vi "Desktop Main.vi"() -> ()   [LabVIEW 2017]
doc: "Demonstrates how to read the button value of the myRIO from the Shared Variable node."
panel:
  out "Boolean 2":bool
  out "error out":errorcluster
  in  "Stop":bool
  # "Overview: Demonstrates how to read the button value of the myRIO from the Shared Variable node.\nInstructions:\n1. Ensure RT Main.vi is already running.\n2. Run this VI. \n3. Press the user button on the myRIO device as many times as you want and observe the value changes of the Button indicator on this VI.\n4. Click Stop to stop this VI."
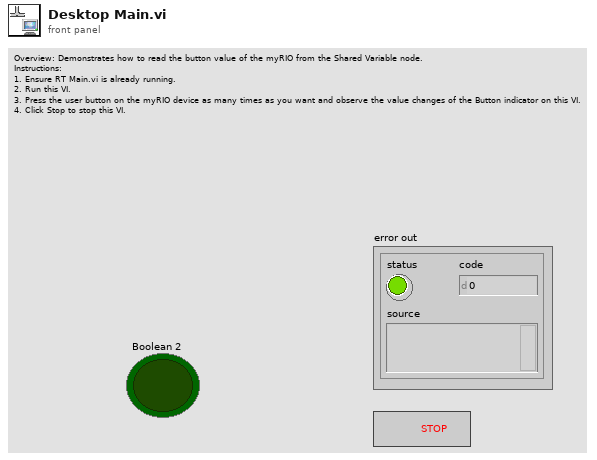
[diagram p1: front panel]
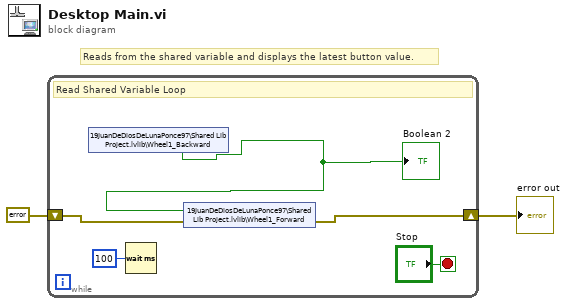
[diagram p0: block diagram]
diagram:
  # "Reads from the shared variable and displays the latest button value."
  n1 = while {
    shift-right: [w4] -> w1
    shift-left: errorcluster {"status"=FALSE, "code"=0, "source"=""} ("error in (no error)") -> [w5]
    stop <- "Stop" stop-if-true
    # "Read Shared Variable Loop"
    n2 = shared-variable "19JuanDeDiosDeLunaPonce97\\Shared Lib Project.lvlib\\Wheel1_Backward"() -> (w3:bool)  [unwired: 1 in, 1 out]
    "Boolean 2" <- w3
    n3 = Wait (ms)(milliseconds to wait=u32 100) -> ()  [unwired: 1 out]
    n4 = shared-variable "19JuanDeDiosDeLunaPonce97\\Shared Lib Project.lvlib\\Wheel1_Forward"(w3, error in=w5) -> (error out=w4:errorcluster)
  }
  "error out" <- w1
